vi "Create Standard Waveform.vi"() -> (2 "Waveform Created?":bool, 3 "Output Waveform":waveform(dbl))   [LabVIEW 2021]
uses:
  <vilib>/Analysis/NI_AALBase.lvlib
  <vilib>/Analysis/1siggen.llb/Ramp Pattern by Samples.vi
panel:
  in  "Suggest Naming?":bool=TRUE
  in  "Waveform Name":string
  in  "Cancel":bool
  in  "OK":bool
  out "Actual Sample Size":i32
  out "Actual Duration (s)":dbl format="%#_6p"
  out "Waveform Preview":waveform(dbl)(graph)
  in  "Sample Rate (Hz)":dbl=10000000.0 min=0.0 format="%#_6p"
  in  "Config Type":enum32{"Periodic", "Ramp", "DC"}(tab)
  in  "Number of Cycles":u32=1 min=1
  in  "Frequency (Hz)":dbl=10000.0 format="%#_6p"
  in  "Amplitude":dbl=1.0
  in  "Ramp Start":dbl
  in  "Ramp Stop":dbl=1.0
  in  "Length (s)":dbl=0.001 format="%#_6p"
  in  "DC Value":dbl format="%#_6p"
  in  "Duration (s)":dbl=0.001 format="%#_6p"
  in  "Waveform Type":i32(listbox)
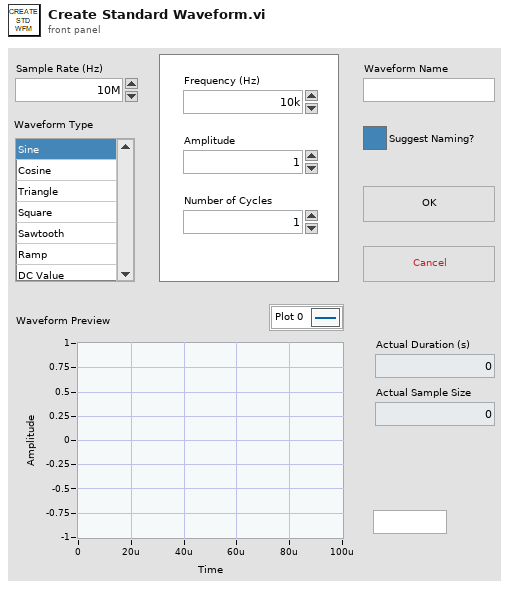
[diagram p1: front panel]
types:
  T1 = enum16{"Ready", "Update Wfm", "Suggest Name Update"}
  T2 = cluster{"Waveform Type":u16, "Amplitude":dbl, "# of Points":u32}
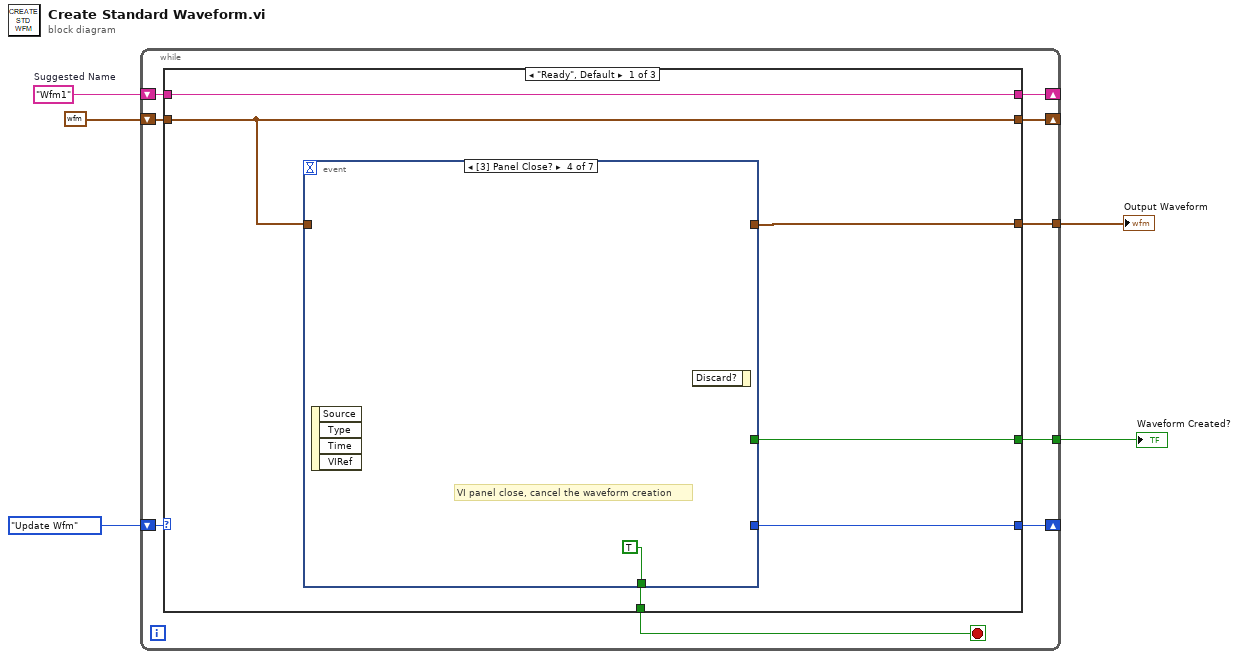
[diagram p0: block diagram]
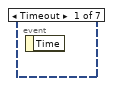
[diagram p2: hidden frame]
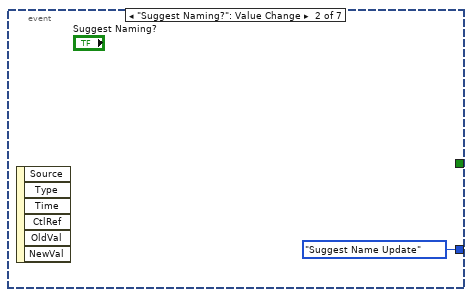
[diagram p3: hidden frame]
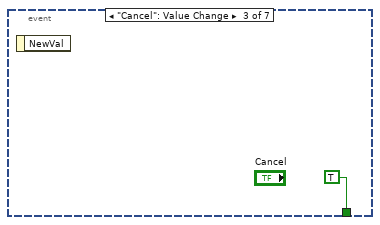
[diagram p4: hidden frame]
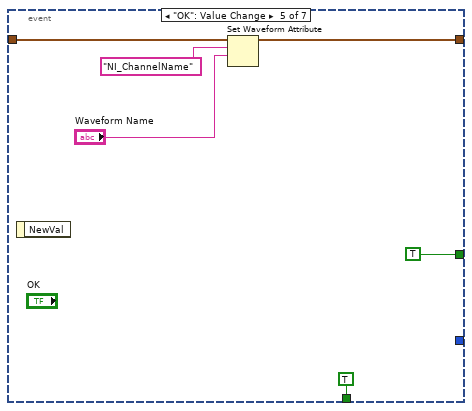
[diagram p5: hidden frame]
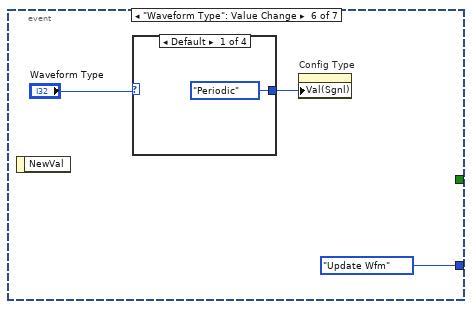
[diagram p6: hidden frame]
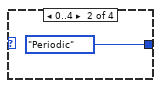
[diagram p7: hidden frame]
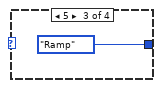
[diagram p8: hidden frame]
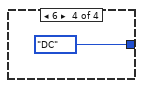
[diagram p9: hidden frame]
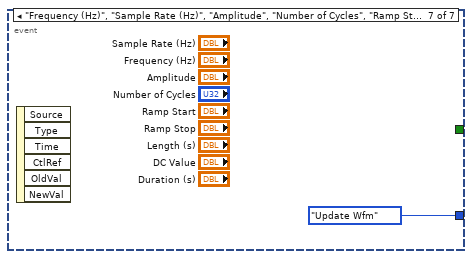
[diagram p10: hidden frame]
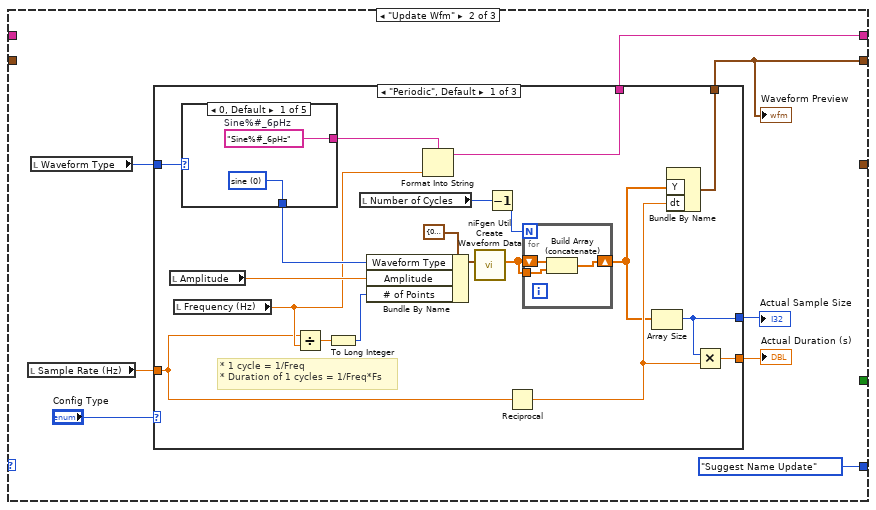
[diagram p11: hidden frame]
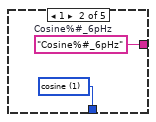
[diagram p12: hidden frame]
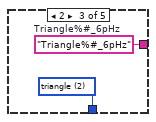
[diagram p13: hidden frame]
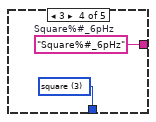
[diagram p14: hidden frame]
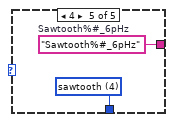
[diagram p15: hidden frame]
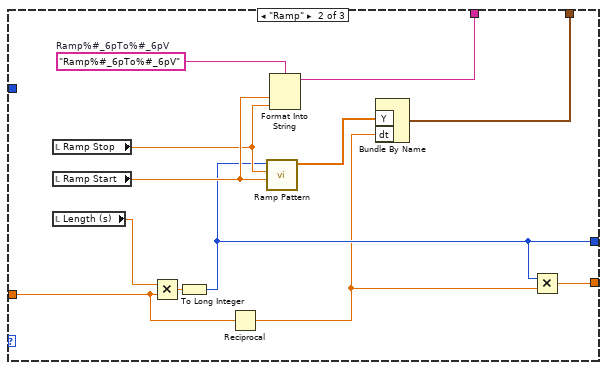
[diagram p16: hidden frame]
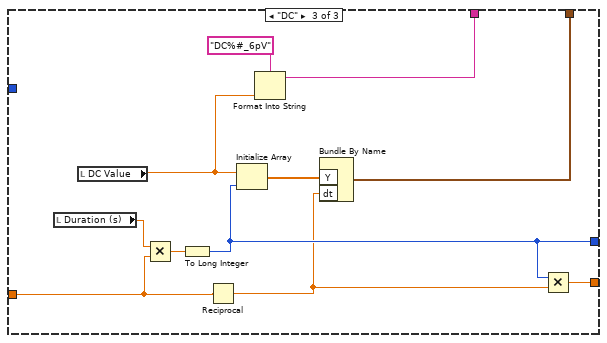
[diagram p17: hidden frame]
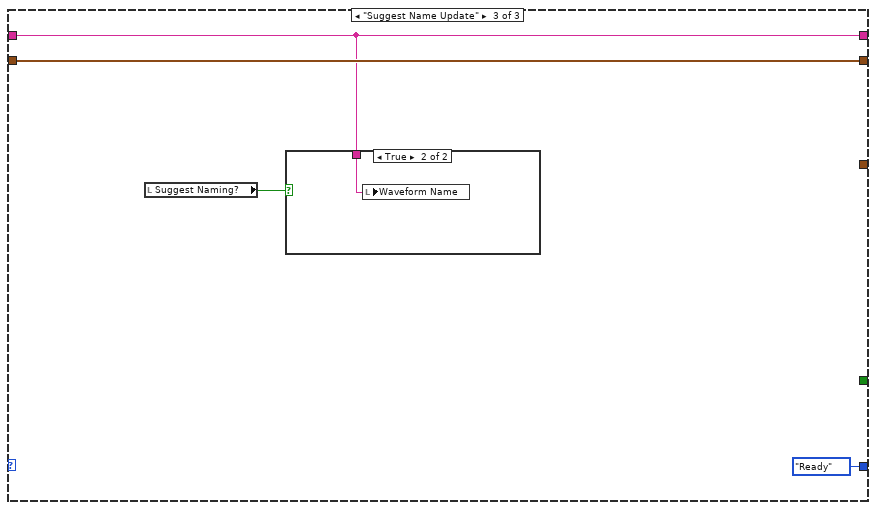
[diagram p18: hidden frame]
diagram:
  w3 = "Wfm1"  # Suggested Name
  n1 = while {
    tunnel: [w13] -> w5
    shift-right: [w11] -> _
    shift-left: T1."Update Wfm" -> [w12]
    shift-right: [w9] -> _
    shift-left: w3 -> [w10]
    shift-right: [w7] -> _
    shift-left: waveform(dbl) {"t0"=timestamp(0 s since 1904-01-01), "dt"=1.0, "Y"=[]} ("Output Waveform") -> [w8]
    tunnel: [w6] -> w1
    stop <- w14 stop-if-true
    n2 = case shown="\"Ready\", Default" w12 {
      tunnel: [w20 _ _] -> w14
      tunnel: [w19 _ _] -> w13
      tunnel: [w18 T1."Suggest Name Update" T1."Ready"] -> w11
      tunnel: w10 -> [w17 _ w102]
      tunnel: [w17 w42 w102] -> w9
      tunnel: w8 -> [w16 _ w104]
      tunnel: [w16 w40 w104] -> w7
      tunnel: [w15 _ _] -> w6
      frame "Ready", Default {
        n3 = event shown="[3] Panel Close?" {
          selector: _ -> [_ _ _ _ _ _ _]
          dyn-events: _ -> [_ _ _ _ _ _ _]
          timeout: _ -> [_ _ _ _ _ _ _]
          tunnel: [_ _ TRUE TRUE TRUE _ _] -> w20
          tunnel: [_ _ _ _ TRUE _ _] -> w19
          tunnel: [_ T1."Suggest Name Update" _ _ _ T1."Update Wfm" T1."Update Wfm"] -> w18
          tunnel: w16 -> [_ _ _ _ w27 _ _]
          tunnel: [_ _ _ _ w24 _ _] -> w15
          event Timeout {
            n4 = event-data() -> ()  [unwired: 1 in, 1 out]
          }
          event "Suggest Naming?": Value Change {
            n5 = event-data() -> ()  [unwired: 1 in, 6 out]
          }
          event "Cancel": Value Change {
            n6 = event-data() -> ()  [unwired: 1 in, 1 out]
          }
          event Panel Close? {
            # "VI panel close, cancel the waveform creation"
            n7 = event-data() -> ()  [unwired: 1 in, 4 out]
            n8 = event-data() -> ()  [unwired: 2 in, 1 out]
          }
          event "OK": Value Change {
            n9 = event-data() -> ()  [unwired: 1 in, 1 out]
            n10 = Set Waveform Attribute(5:"Waveform Name", 6:"NI_ChannelName" ("name"), 7:w27) -> (3:w24:waveform(dbl))  [unwired: 1 in, 2 out]
          }
          event "Waveform Type": Value Change {
            n11 = event-data() -> ()  [unwired: 1 in, 1 out]
            n12 = case shown="Default" "Waveform Type" {
              tunnel: [enum32{"Periodic", "Ramp", "DC"}."Periodic" ("Value (Signaling)") enum32{"Periodic", "Ramp", "DC"}."Periodic" ("Value (Signaling)") enum32{"Periodic", "Ramp", "DC"}."Ramp" ("Value (Signaling)") enum32{"Periodic", "Ramp", "DC"}."DC" ("Value (Signaling)")] -> w32
              frame Default {
              }
              frame 0..4 {
              }
              frame 5 {
              }
              frame 6 {
              }
            }
            n13 = property on="Config Type" class="TabCtl (strict)"("Val(Sgnl)"=w32) -> ()  [unwired: 2 in, 2 out]
          }
          event "Frequency (Hz)", "Sample Rate (Hz)", "Amplitude", "Number of Cycles", "Ramp Start", "Ramp Stop", "Length (s)", "Duration (s)", "DC Value": Value Change {
            n14 = event-data() -> ()  [unwired: 1 in, 6 out]
          }
        }
      }
      frame "Update Wfm" {
        n15 = local read "Sample Rate (Hz)"() -> (w44:dbl)
        n16 = local read "Waveform Type"() -> (w43:i32)
        n17 = case shown="\"Periodic\", Default" "Config Type" {
          tunnel: w44 -> [w51 w87 w99]
          tunnel: w43 -> [w61 _ _]
          tunnel: [w58 w81 w90] -> w42
          tunnel: [w59 w85 w96] -> w40
          tunnel: [w46 w79 w94] -> w39
          tunnel: [w53 w80 w95] -> w38
          frame "Periodic", Default {
            # "* 1 cycle = 1/Freq\n* Duration of 1 cycles = 1/Freq*Fs"
            n18 = local read "Amplitude"() -> (w62:dbl)
            n19 = local read "Frequency (Hz)"() -> (w56:dbl)
            n20 = case shown="0, Default" w61 {
              tunnel: [w69 w71 w73 w75 w77] -> w60
              tunnel: [w68 w70 w72 w74 w76] -> w57
              frame 0, Default {
                w68 = "Sine%#_6pHz"  # Sine%#_6pHz
                w69 = u16 0 items=["sine", "cosine", "triangle", "square", "sawtooth", "increasing ramp", "decreasing ramp", "DC Value"] ("Waveform Type")
              }
              frame 1 {
                w70 = "Cosine%#_6pHz"  # Cosine%#_6pHz
                w71 = u16 1 items=["sine", "cosine", "triangle", "square", "sawtooth", "increasing ramp", "decreasing ramp", "DC Value"] ("Waveform Type")
              }
              frame 2 {
                w72 = "Triangle%#_6pHz"  # Triangle%#_6pHz
                w73 = u16 2 items=["sine", "cosine", "triangle", "square", "sawtooth", "increasing ramp", "decreasing ramp", "DC Value"] ("Waveform Type")
              }
              frame 3 {
                w74 = "Square%#_6pHz"  # Square%#_6pHz
                w75 = u16 3 items=["sine", "cosine", "triangle", "square", "sawtooth", "increasing ramp", "decreasing ramp", "DC Value"] ("Waveform Type")
              }
              frame 4 {
                w76 = "Sawtooth%#_6pHz"  # Sawtooth%#_6pHz
                w77 = u16 4 items=["sine", "cosine", "triangle", "square", "sawtooth", "increasing ramp", "decreasing ramp", "DC Value"] ("Waveform Type")
              }
            }
            n21 = Divide(x=w51, y=w56) -> (x/y=w52:dbl)
            n22 = To Long Integer(number=w52) -> (32bit integer=w55:i32)
            n23 = local read "Number of Cycles"() -> (w49:u32)
            n24 = Bundle By Name(cluster=T2 {"Waveform Type"=0, "Amplitude"=1.0, "# of Points"=256} ("Waveform"), "Waveform Type"=w60, "Amplitude"=w62, "# of Points"=w55) -> (w63:T2)
            n25 = Format Into String(format string=w57, w56) -> (resulting string=w58:string)  [unwired: 2 in, 1 out]
            n26 = call <instrlib>:"niFgen Util Create Waveform Data.vi"("Waveform"=w63) -> ("Waveform Data"=w50:dbl[])  [unwired: 10 in]
            n27 = Decrement(x=w49) -> (x-1=w48:u32)
            n28 = Reciprocal(x=w51) -> (1/x=w54:dbl)
            n29 = for {
              N: w48 -> [_]
              shift-right: [w66] -> w47
              shift-left: w50 -> [w67]
              tunnel: w50 -> [w65]
              n30 = Build Array (concatenate)(w67, w65) -> (w66:dbl[])
            }
            n31 = Array Size(array=w47) -> (size(s)=w46:i32)
            n32 = Bundle By Name("Y"=w47, "dt"=w54) -> (w59:waveform(dbl))  [unwired: 1 in]
            n33 = Multiply(x=w46, y=w54) -> (x*y=w53:dbl)
          }
          frame "Ramp" {
            w84 = "Ramp%#_6pTo%#_6pV"  # Ramp%#_6pTo%#_6pV
            n34 = local read "Ramp Stop"() -> (w82:dbl)
            n35 = local read "Ramp Start"() -> (w83:dbl)
            n36 = local read "Length (s)"() -> (w89:dbl)
            n37 = Multiply(x=w89, y=w87) -> (x*y=w88:dbl)
            n38 = To Long Integer(number=w88) -> (32bit integer=w79:i32)
            n39 = Reciprocal(x=w87) -> (1/x=w78:dbl)
            n40 = call-poly <vilib>:"Ramp Pattern.vi"("start"=w83, "end"=w82, "samples"=w79) -> ("Ramp Pattern"=w86:dbl[])  [unwired: 7 in, 1 out]
            n41 = Format Into String(format string=w84, w83, w82) -> (resulting string=w81:string)  [unwired: 2 in, 1 out]
            n42 = Bundle By Name("Y"=w86, "dt"=w78) -> (w85:waveform(dbl))  [unwired: 1 in]
            n43 = Multiply(x=w79, y=w78) -> (x*y=w80:dbl)
          }
          frame "DC" {
            n44 = local read "Duration (s)"() -> (w100:dbl)
            n45 = local read "DC Value"() -> (w91:dbl)
            n46 = Multiply(x=w100, y=w99) -> (x*y=w98:dbl)
            n47 = To Long Integer(number=w98) -> (32bit integer=w94:i32)
            n48 = Reciprocal(x=w99) -> (1/x=w93:dbl)
            n49 = Initialize Array(w91, w94) -> (w97:dbl[])
            n50 = Format Into String(format string="DC%#_6pV", w91) -> (resulting string=w90:string)  [unwired: 2 in, 1 out]
            n51 = Bundle By Name("Y"=w97, "dt"=w93) -> (w96:waveform(dbl))  [unwired: 1 in]
            n52 = Multiply(x=w94, y=w93) -> (x*y=w95:dbl)
          }
        }
        "Waveform Preview" <- w40
        "Actual Duration (s)" <- w38
        "Actual Sample Size" <- w39
      }
      frame "Suggest Name Update" {
        n53 = local read "Suggest Naming?"() -> (w103:bool)
        n54 = case shown="True" w103 {
          tunnel: w102 -> [_ w105]
          frame False {
          }
          frame True {
            n55 = local write "Waveform Name"(w105) -> ()
          }
        }
      }
    }
  }
  "Waveform Created?" <- w5
  "Output Waveform" <- w1
